vi "Search 1D Array for ALL matches.vi"(8 "error in (no error)":errorcluster, 10 "Se4arch string":string, 11 "1D String Array":string[](array[string])) -> (0 "error out":errorcluster, 3 "Found positions Array":i32[](array[numeric]))   [LabVIEW 2012]
doc: "SciScan 1.2 160622"
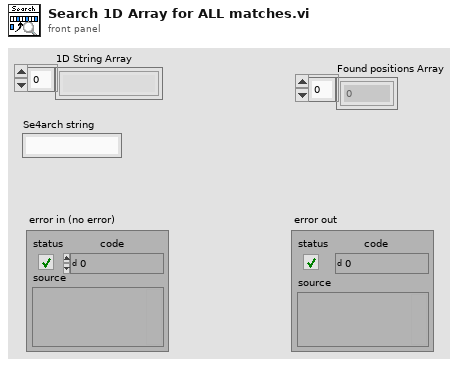
[diagram p1: front panel]
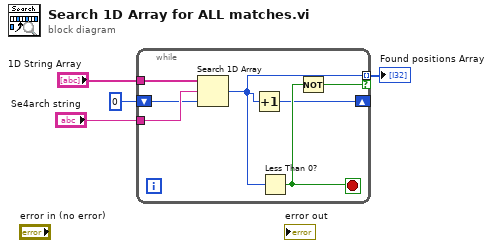
[diagram p0: block diagram]
diagram:
  n1 = while {
    tunnel: "Se4arch string" -> [w11]
    tunnel: "1D String Array" -> [w10]
    tunnel: [w6] -> w2 mode=indexing if=w8
    shift-right: [w5] -> _
    shift-left: 0 ("index of element") -> [w7]
    stop <- w9 stop-if-true
    n2 = Search 1D Array(1D array=w10, element=w11, start index (0)=w7) -> (index of element=w6:i32)
    n3 = Increment(x=w6) -> (x+1=w5:i32)
    n4 = Less Than 0?(x=w6) -> (x < 0?=w9:bool)
    n5 = Not(x=w9) -> (.not. x?=w8:bool)
  }
  "Found positions Array" <- w2
